vi "_wmg_whetherItemsEmpty.vi"(1 "Input":i32[][](array[numeric])) -> (0 "bool":bool)   [LabVIEW 2011]
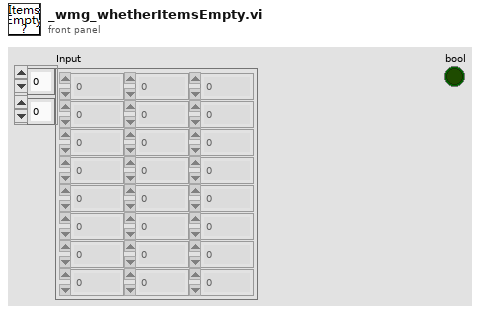
[diagram p1: front panel]
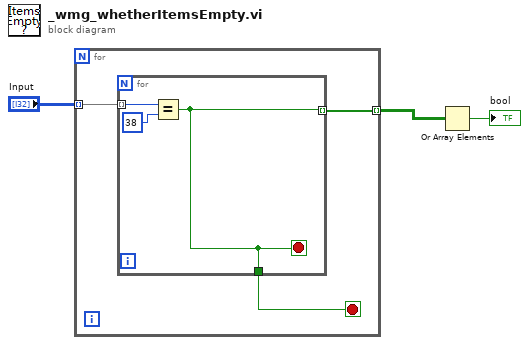
[diagram p0: block diagram]
diagram:
  n1 = for "For循环" {
    tunnel: "Input" -> [w6] mode=indexing
    tunnel: [w5] -> w2 mode=indexing
    stop <- w4 stop-if-true
    n2 = for "For循环" {
      tunnel: w6 -> [w9] mode=indexing
      tunnel: [w7] -> w5 mode=indexing
      tunnel: [w7] -> w4
      stop <- w7 stop-if-true
      n3 = Equal?(x=w9, y=38) -> (x = y?=w7:bool)
    }
  }
  n4 = Or Array Elements(Boolean array=w2) -> (logical OR=→"bool":bool)
